vi "BUILD_uninstall.vi"() -> ()   [LabVIEW 2013]
panel:
  out "error out":errorcluster
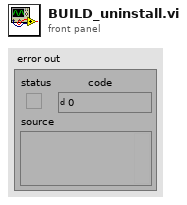
[diagram p1: front panel]
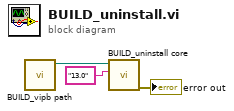
[diagram p0: block diagram]
diagram:
  n1 = call "BUILD_vipb path.vi"() -> ("appended path"=w1:path)  [unwired: 11 in]
  n2 = call "BUILD_uninstall core.vi"("LabVIEW Version"="13.0", "appended path"=w1) -> ("error out"=→"error out":errorcluster)  [unwired: 9 in]
